vi "nanocal -- generate 3D curvature ellipsoid --  V5.vi"(0 "parameter keys IN":T2[](array[typedef])=[enum."ζ", enum."τ1", enum."τS", enum."τN", enum."τC", enum."κ0"], 5 "parameter tensor order IN":map{i32, T2}(c390), 7 "parameters IN":map{T2, dbl}(c390), 9 "data IN":T3={"dz/dω  (sec/rad)"=[], "z "=[1.7183506006211996e-05-0.0001154032788780638i, 1.7124360968751133e-05-0.0001154114779288915i, 1.7049104347380084e-05-0.00011541542942613611i, 1.700437896335042e-05-0.00011541749156201827i, 1.6984579723285106e-05-0.00011542204741013496i, 1.702277369054923e-05-0.00011543195548892015i, 1.713094025845651e-05-0.00011543928112855599i, 1.734249707866828e-05-0.00011543960094139092i, 1.768320429215342e-05-0.0001154245402225022i, 1.8195281152538477e-05-0.00011538335923575508i, 1.8917228661806973e-05-0.00011530288392402138i, 1.9897834564883332e-05-0.00011516640933089982i, 2.154104046962704e-05-0.0001148906117047364i, 2.3247799321765792e-05-0.00011455940834964969i, 2.5364678450551808e-05-0.00011410149936074356i, 2.8645788781885885e-05-0.00011331572480450341i, 3.204749554800641e-05-0.00011242961468546203i, 3.783559691555022e-05-0.00011080033368711338i, 4.245015867332296e-05-0.00010941815048749576i, 4.909131821431355e-05-0.0001073312840925185i, 5.511821898441184e-05-0.00010535829212367013i, 6.178843506022867e-05-0.00010310289174359778i, 7.1079604965352e-05-9.985157907779013e-05i, 7.922304381453334e-05-9.690255343156676e-05i, 8.814778883893872e-05-9.35627973091444e-05i, 9.806709148886077e-05-8.971246458508318e-05i, 0.00011119043245647465-8.437841897470898e-05i, 0.00012253184919712196-7.953180105990741e-05i, 0.00013777724317049346-7.26422052575784e-05i, 0.0001508081004573332-6.638511645494567e-05i, 0.00016547294918783876-5.890291826790314e-05i, 0.00018003847596605868-5.097295421607585e-05i, 0.00019518361086534857-4.2160672625888326e-05i, 0.00021134179818259658-3.207632261667366e-05i, 0.0002372041782935464-1.434566976209705e-05i, 0.00025518143132024254-7.65423157605567e-07i, 0.0002835129702467886+2.297908707067173e-05i, 0.0003060118087631287+4.414715126576145e-05i, 0.00032860772064336976+6.780161699354136e-05i, 0.0003492674091322389+9.188627597766353e-05i, 0.00037498324855458583+0.0001258445655672888i, 0.00040021078021115026+0.00016463936720210011i, 0.00041969942568205823+0.0001996255883353531i, 0.00044367338947118773+0.00025154867300893595i, 0.0004634793607238068+0.0003068834938295352i, 0.00047921028781215815+0.00036805191402776324i, 0.0004880906353641744+0.00042166295770603194i, 0.0004932212623741357+0.0004947057496862386i, 0.000491476456593048+0.0005562791342814882i, 0.000480893803992059+0.0006363872629062725i, 0.0004535995818650303+0.0007373086546111893i, 0.000417087772881063+0.0008226852134031236i, 0.0003564148692854789+0.0009214817173403453i, 0.0003049201646356487+0.0009841224100520793i, 0.00021260191240459413+0.0010684135492785532i, 0.00011714858948470126+0.001130293664798013i, 1.675457544365132e-05+0.0011752384955043165i, -6.8674075405897e-05+0.0012001399159748158i, -0.000156473047607305+0.0012143601357779102i, -0.00026709373934749337+0.0012167952520739987i, -0.0003544271565676041+0.001206585218500233i, -0.00047937600197311275+0.0011721904461218277i, -0.0006086290582260493+0.0011080263068835828i, -0.0007031877411848573+0.0010369948237613604i, -0.0007564526901441745+0.0009845652865779295i, -0.000802489180995596+0.0009292050493656664i, -0.0008414596018105983+0.0008721985101652608i, -0.0008809346482248761+0.0008000538120167723i, -0.0009073902840241921+0.0007382113118499092i, -0.0009264953054508651+0.000680980624166274i, -0.0009405659412141811+0.0006247883223244968i, -0.000951649722530156+0.0005564170049287236i, -0.0009557485581057351+0.0005027508202624884i, -0.0009558464741053665+0.0004515634249715623i, -0.0009509110176922098+0.0003899637122391104i, -0.0009411315169847015+0.00033238768338539245i, -0.0009303400913929496+0.0002890952314710416i, -0.0009171113529290538+0.00024772942260094455i, -0.0009022111527275027+0.00020961974320628598i, -0.0008813746494947608+0.00016554205395646727i, -0.0008581837971946129+0.00012481593212717478i, -0.0008372063466683705+9.328565348151487e-05i, -0.0008165626610594428+6.595676342721183e-05i, -0.0007901155435838691+3.51376371228606e-05i, -0.0007682834352800848+1.2585785624721776e-05i, -0.000746231015527196-7.956667433689733e-06i, -0.0007238798463130141-2.6771164006128246e-05i, -0.0007015567569177018-4.3779400880525094e-05i, -0.000679301954671598-5.9154880569231366e-05i, -0.0006572001413831251-7.301304884663801e-05i, -0.000629855254567978-8.838260380910578e-05i, -0.0006083942229188815-9.917719243438264e-05i, -0.0005768631156754208-0.00011317657292622015i, -0.0005562177438951648-0.00012121832857134644i, -0.0005359092039599222-0.00012831021292074535i, -0.0005145186443378148-0.00013494179211461784i, -0.0004951602053444319-0.00014023403510992087i, -0.00047624970229075174-0.00014478034103386663i, -0.0004577401041527736-0.00014865456703421655i, -0.00043519037796120065-0.00015262867452433312i], "ω (rad/sec)"=[32012.991918577427, 32390.261658505893, 32466.39798177853, 32499.14340521798, 32517.39286113775, 32529.046092051318, 32537.14525712326, 32543.111142615544, 32547.696343954158, 32551.33675949651, 32554.302325209504, 32556.769142360055, 32558.856995237307, 32560.650202739795, 32562.209843476354, 32563.58125099723, 32564.7987833122, 32565.88895894197, 32566.872575330308, 32567.766175404246, 32568.583086316496, 32569.334166794306, 32570.02835688638, 32570.673085530187, 32571.274580490695, 32571.838104118455, 32572.36813539066, 32572.868514009202, 32573.342552524307, 32573.793126289274, 32574.222746575288, 32574.633618125405, 32575.027687968828, 32575.40668442971, 32575.772149741057, 32576.12546690325, 32576.467883345118, 32576.800529469096, 32577.124435064776, 32577.440543590797, 32577.749724325146, 32578.052781957467, 32578.35046682089, 32578.643482565894, 32578.932492128843, 32579.218126471686, 32579.500987779396, 32579.781656707495, 32580.06069600583, 32580.338656060805, 32580.616078519142, 32580.89350097748, 32581.171461032456, 32581.45050033079, 32581.73116925889, 32582.0140305666, 32582.29966469628, 32582.58867447239, 32582.88169000423, 32583.179375080817, 32583.48243271314, 32583.791613234323, 32584.10772197351, 32584.43162756919, 32584.764273480003, 32585.106690135035, 32585.460007297228, 32585.825472395412, 32586.204468856296, 32586.59853891288, 32587.009410462997, 32587.439030535847, 32587.889604513977, 32588.363642815923, 32588.86402143446, 32589.39405291983, 32589.957576334426, 32590.559071508098, 32591.203800151903, 32591.897990030815, 32592.64907072179, 32593.46598163404, 32594.359581707977, 32595.343197883154, 32596.433373726086, 32597.650906041054, 32599.022313348767, 32600.58195429849, 32602.375161800977, 32604.46301467823, 32606.929831615616, 32609.895397541775, 32613.535812870963, 32618.12101442274, 32624.086899701866, 32632.186064986967, 32643.839295900536, 32662.088751820305, 32694.834175046595, 32770.97049853239]}, 11 "errors IN":T1={"one"=enum."τ1", "two"=enum."τS", "sigmaone"=enum."στ1", "sigmatwo"=enum."στS", "three"=enum."τN", "sigmathree"=enum."στN", "pars & errors"={}, "T22 factor"=5.0, "CN2 factor"=0.1, "δG/G"=0.5535743588970453, "noise T"=0.1, "Δlogs"=[3.0, 1.0], "Δlog ηs"=[4.618033988749895, 2.381966011250105]} {"Δlog ηs" format="%#_2f"; "Δlogs" format="%#_2f"; "noise T" format="%#_3f"; "δG/G" format="%#_3f"; "CN2 factor" min=0.0 max=0.3 step=1e-06 scale=0.01..1.0 scale format="%#_2f"; "T22 factor" min=0.0 max=0.3 step=1e-06 scale=0.1..20.0 scale format="%#_2f"}, 12 "newton parameters":T4={"method"=enum."ignore", "weighting"=enum."dω √(|dz/dω|)", "PID-P"=0.009761510697263134, "PID-I"=5} {"PID-P" scale=1e-09..10.0 scale format="%#_3p"}) -> (15 "errors pair OUT":T1={"one"=enum."τ1", "two"=enum."τS", "sigmaone"=enum."στ1", "sigmatwo"=enum."στS", "three"=enum."τN", "sigmathree"=enum."στN", "pars & errors"={}, "T22 factor"=5.0, "CN2 factor"=0.1, "δG/G"=0.5535743588970453, "noise T"=0.1, "Δlogs"=[3.0, 1.0], "Δlog ηs"=[4.618033988749895, 2.381966011250105]} {"Δlog ηs" format="%#_2f"; "Δlogs" format="%#_2f"; "noise T" format="%#_3f"; "δG/G" format="%#_3f"; "CN2 factor" min=0.0 max=0.3 step=1e-06 scale=0.01..1.0 scale format="%#_2f"; "T22 factor" min=0.0 max=0.3 step=1e-06 scale=0.1..20.0 scale format="%#_2f"})   [LabVIEW 2021]
uses:
  3-lorentzian-parameters.ctl
  nanocal -- gradient descent -- parameters.ctl
  linear regression type.ctl
  nanocal-goodness-weighting-strategy.ctl
  nanocal -- gradient descent-- data.ctl
  3D curvature triplet control -- V2.ctl
  nanocal generate curvature ellipse -- action.ctl
  3-lorentzian-heat-response action.ctl
  array -- 3-finitediff.vi
  5-lorentzian-heat-response -- analytic derivatives -- grad and curvature -- V6.vi
  <vilib>/Analysis/Matrix/Numeric/Conversions/Array To Matrix.vi
  <vilib>/Analysis/Matrix/Numeric/Conversions/Array To Matrix - RA2.vi
  <vilib>/Analysis/baseanly.llb/Inverse Matrix.vi
  <vilib>/Analysis/baseanly.llb/Real Inverse Matrix.vi
  <vilib>/Analysis/Matrix/Numeric/Conversions/Matrix To Array.vi
  <vilib>/Analysis/Matrix/Numeric/Conversions/Matrix To Array - RM.vi
  <vilib>/Analysis/Matrix/Numeric/Conversions/Array To Matrix - RA.vi
  <vilib>/Analysis/7linalg.llb/Solve Linear Equations.vi
  <vilib>/Analysis/7linalg.llb/Solve Linear Equations (multiple right hand).vi
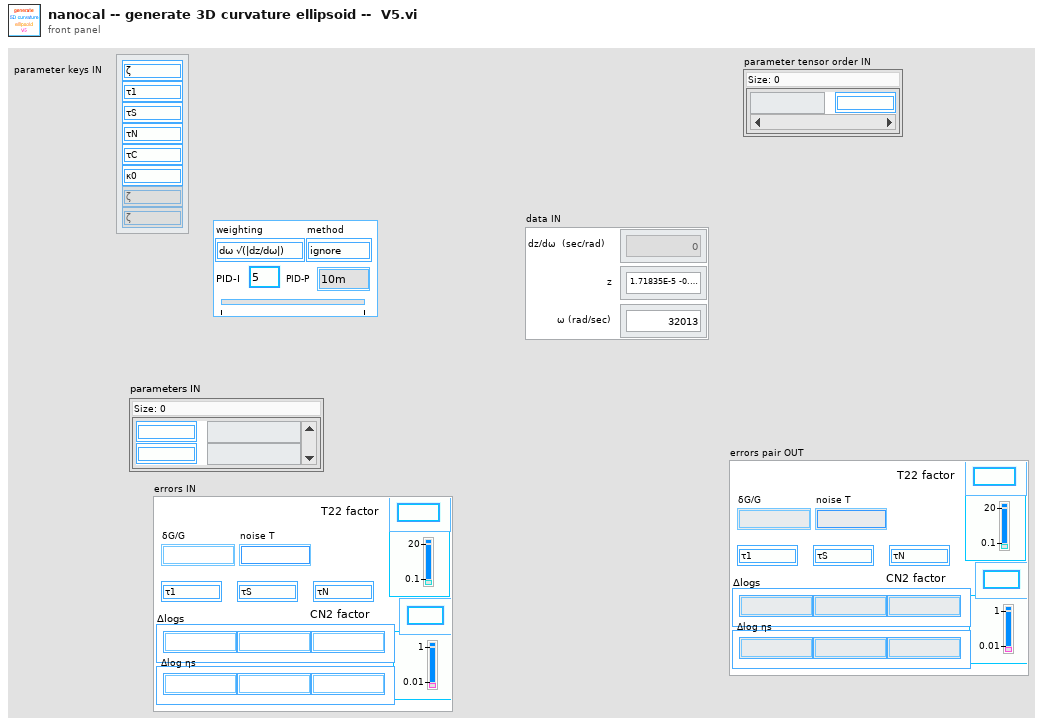
[diagram p1: front panel]
types:
  T1 = typedef "3D curvature triplet control -- V2.ctl" = cluster{"one":T2, "two":T2, "sigmaone":T2, "sigmatwo":T2, "three":T2, "sigmathree":T2, "pars & errors":map{T2, dbl}, "T22 factor":dbl, "CN2 factor":dbl, "δG/G":dbl, "noise T":dbl, "Δlogs":dbl[], "Δlog ηs":dbl[]}
  T2 = typedef "3-lorentzian-parameters.ctl" = enum16{"ζ", "τ1", "τS", "τN", "τC", "κ0", "m1", "m2", "m3", "T (K)", "B (T)", "θ (deg)", "side (S|R)", "set of (B|T)", "Re(offset)", "Im(offset)", "στ1", "στ1-", "στ1+", "στS", "στS-", "στS+", "στN", "στN-", "στN+", "τ11", "τ12", "τ21", "τ22", "τN1", "τN2", "σηlogτ1", "σηlogτS", "σηlogτN", "σlogτ1", "σlogτS", "σlogτN", "σητ1", "σητS", "σητN", "noiseT"}
  T3 = typedef "nanocal -- gradient descent-- data.ctl" = cluster{"dz/dω  (sec/rad)":cdb[], "z ":cdb[], "ω (rad/sec)":dbl[]}
  T4 = typedef "nanocal -- gradient descent -- parameters.ctl" = cluster{"method":T5, "weighting":T6, "PID-P":dbl, "PID-I":i32}
  T5 = typedef "linear regression type.ctl" = enum16{"ignore", "gradient", "newton"}
  T6 = typedef "nanocal-goodness-weighting-strategy.ctl" = enum16{"dω", "dω √(|dz/dω|)", "dω |dz/dω|", "phase", "andreas", "sum", "anti-andr", "ark"}
  T7 = typedef "nanocal generate curvature ellipse -- action.ctl" = enum16{"errors-log", "errors-linear"}
  T8 = typedef "3-lorentzian-heat-response action.ctl" = enum16{"calc R", "create string", "calc m1m2m3", "dζ", "dT1", "dτS", "dτN", "dτC", "d-all", "dκ0", "T(K)", "m1", "m2", "m3", "parse string", "θ (deg)", "B (T)", "onlygrads", "newton", "create emty string", "simple2nd", "calc R2", "ScalarProd", "ScalarProd-diff", "nothing", "ScalarProd-eta", "tolog", "ignore", "three2nd", "eta-errors"}
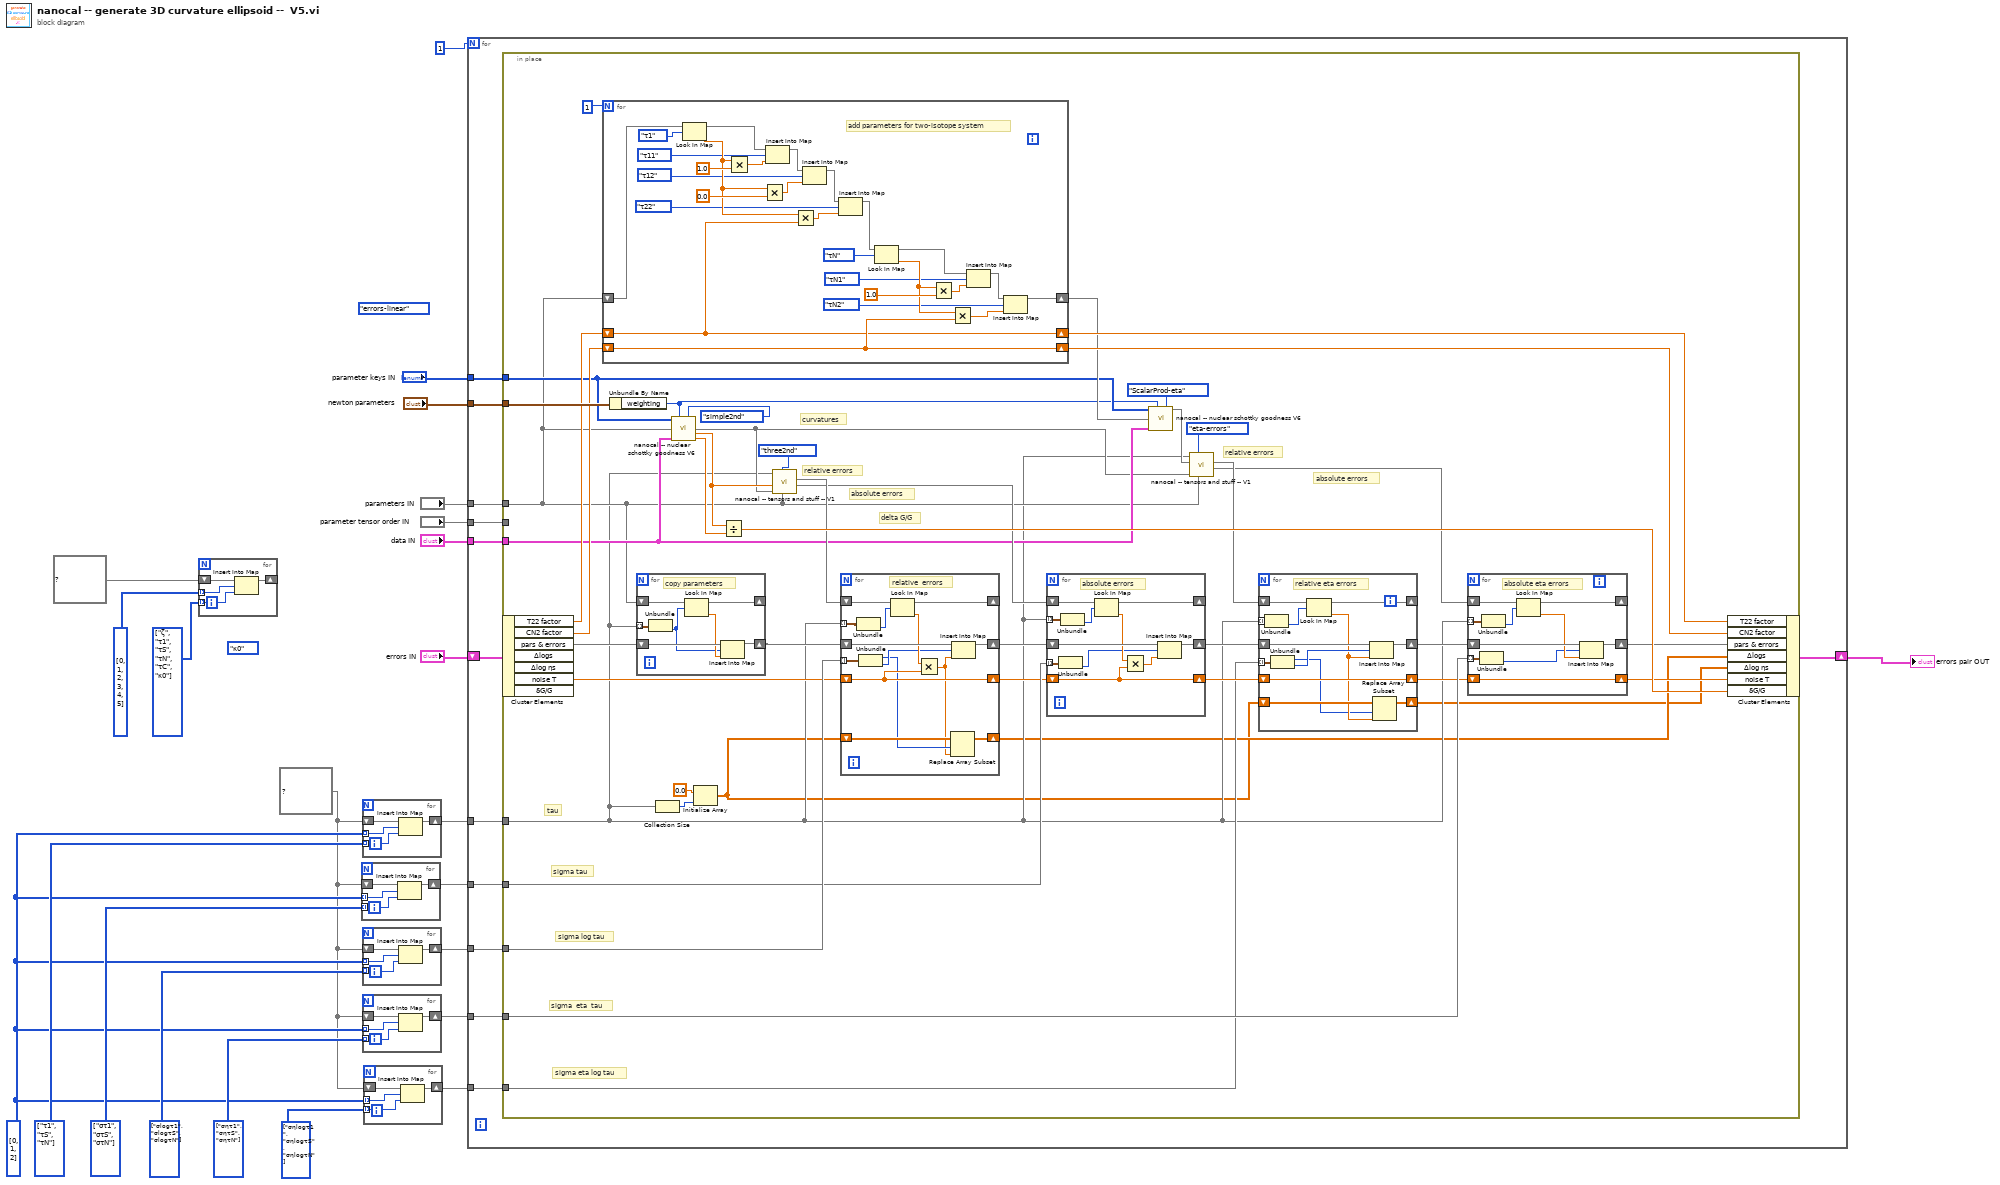
[diagram p0: block diagram]
diagram:
  w4 = T2[] [enum."σηlogτ1", enum."σηlogτS", enum."σηlogτN"] items=["ζ", "τ1", "τS", "τN", "τC", "κ0", "m1", "m2", "m3", "T (K)", "B (T)", "θ (deg)", "side (S|R)", "set of (B|T)", "Re(offset)", "Im(offset)", "στ1", "στ1-", "στ1+", "στS", "στS-", "στS+", "στN", "στN-", "στN+", "τ11", "τ12", "τ21", "τ22", "τN1", "τN2", "σηlogτ1", "σηlogτS", "σηlogτN", "σlogτ1", "σlogτS", "σlogτN", "σητ1", "σητS", "σητN", "noiseT"]
  w9 = T2[] [enum."σlogτ1", enum."σlogτS", enum."σlogτN"] items=["ζ", "τ1", "τS", "τN", "τC", "κ0", "m1", "m2", "m3", "T (K)", "B (T)", "θ (deg)", "side (S|R)", "set of (B|T)", "Re(offset)", "Im(offset)", "στ1", "στ1-", "στ1+", "στS", "στS-", "στS+", "στN", "στN-", "στN+", "τ11", "τ12", "τ21", "τ22", "τN1", "τN2", "σηlogτ1", "σηlogτS", "σηlogτN", "σlogτ1", "σlogτS", "σlogτN", "σητ1", "σητS", "σητN", "noiseT"]
  w10 = T2[] [enum."σητ1", enum."σητS", enum."σητN"] items=["ζ", "τ1", "τS", "τN", "τC", "κ0", "m1", "m2", "m3", "T (K)", "B (T)", "θ (deg)", "side (S|R)", "set of (B|T)", "Re(offset)", "Im(offset)", "στ1", "στ1-", "στ1+", "στS", "στS-", "στS+", "στN", "στN-", "στN+", "τ11", "τ12", "τ21", "τ22", "τN1", "τN2", "σηlogτ1", "σηlogτS", "σηlogτN", "σlogτ1", "σlogτS", "σlogτN", "σητ1", "σητS", "σητN", "noiseT"]
  w11 = T2[] [enum."στ1", enum."στS", enum."στN"] items=["ζ", "τ1", "τS", "τN", "τC", "κ0", "m1", "m2", "m3", "T (K)", "B (T)", "θ (deg)", "side (S|R)", "set of (B|T)", "Re(offset)", "Im(offset)", "στ1", "στ1-", "στ1+", "στS", "στS-", "στS+", "στN", "στN-", "στN+", "τ11", "τ12", "τ21", "τ22", "τN1", "τN2", "σηlogτ1", "σηlogτS", "σηlogτN", "σlogτ1", "σlogτS", "σlogτN", "σητ1", "σητS", "σητN", "noiseT"]
  (unwired) 3-lorentzian-parameters."κ0" ("X selector")
  w3 = i32[] [0, 1, 2]
  w2 = map{i32, T2} {} ("parameters IN")
  w13 = T2[] [enum."τ1", enum."τS", enum."τN"] items=["ζ", "τ1", "τS", "τN", "τC", "κ0", "m1", "m2", "m3", "T (K)", "B (T)", "θ (deg)", "side (S|R)", "set of (B|T)", "Re(offset)", "Im(offset)", "στ1", "στ1-", "στ1+", "στS", "στS-", "στS+", "στN", "στN-", "στN+", "τ11", "τ12", "τ21", "τ22", "τN1", "τN2", "σηlogτ1", "σηlogτS", "σηlogτN", "σlogτ1", "σlogτS", "σlogτN", "σητ1", "σητS", "σητN", "noiseT"]
  w16 = T2[] [enum."ζ", enum."τ1", enum."τS", enum."τN", enum."τC", enum."κ0"] items=["ζ", "τ1", "τS", "τN", "τC", "κ0", "m1", "m2", "m3", "T (K)", "B (T)", "θ (deg)", "side (S|R)", "set of (B|T)", "Re(offset)", "Im(offset)", "στ1", "στ1-", "στ1+", "στS", "στS-", "στS+", "στN", "στN-", "στN+", "τ11", "τ12", "τ21", "τ22", "τN1", "τN2", "σηlogτ1", "σηlogτS", "σηlogτN", "σlogτ1", "σlogτS", "σlogτN", "σητ1", "σητS", "σητN", "noiseT"]
  (unwired) nanocal_generate_curvature_ellipse_--_action."errors-linear" ("Enum")
  n1 = for {
    tunnel: w16 -> [w24] mode=indexing
    shift-right: [w26] -> _
    shift-left: map{i32, T2} {} ("parameters IN") -> [w27]
    tunnel: i32[] [0, 1, 2, 3, 4, 5] -> [w25] mode=indexing
    n2 = Insert Into Map(map in=w27, key=w25, value=w24) -> (map out=w26:map{i32, T2})  [unwired: 2 out]
  }
  n3 = for {
    tunnel: w11 -> [w28] mode=indexing
    shift-right: [w30] -> w7
    shift-left: w2 -> [w31]
    tunnel: w3 -> [w29] mode=indexing
    n4 = Insert Into Map(map in=w31, key=w29, value=w28) -> (map out=w30:map{i32, T2})  [unwired: 2 out]
  }
  n5 = for {
    tunnel: w13 -> [w32] mode=indexing
    shift-right: [w34] -> w12
    shift-left: w2 -> [w35]
    tunnel: w3 -> [w33] mode=indexing
    n6 = Insert Into Map(map in=w35, key=w33, value=w32) -> (map out=w34:map{i32, T2})  [unwired: 2 out]
  }
  n7 = for {
    tunnel: w9 -> [w36] mode=indexing
    shift-right: [w38] -> w8
    shift-left: w2 -> [w39]
    tunnel: w3 -> [w37] mode=indexing
    n8 = Insert Into Map(map in=w39, key=w37, value=w36) -> (map out=w38:map{i32, T2})  [unwired: 2 out]
  }
  n9 = for {
    tunnel: w10 -> [w40] mode=indexing
    shift-right: [w42] -> w6
    shift-left: w2 -> [w43]
    tunnel: w3 -> [w41] mode=indexing
    n10 = Insert Into Map(map in=w43, key=w41, value=w40) -> (map out=w42:map{i32, T2})  [unwired: 2 out]
  }
  n11 = for {
    tunnel: w4 -> [w44] mode=indexing
    shift-right: [w46] -> w1
    shift-left: w2 -> [w47]
    tunnel: w3 -> [w45] mode=indexing
    n12 = Insert Into Map(map in=w47, key=w45, value=w44) -> (map out=w46:map{i32, T2})  [unwired: 2 out]
  }
  n13 = for {
    N: 1 -> [_]
    tunnel: "newton parameters" -> [w59]
    tunnel: "data IN" -> [w58]
    tunnel: "parameters IN" -> [w57]
    tunnel: "parameter keys IN" -> [w56]
    tunnel: "parameter tensor order IN" -> [w55]
    shift-right: [w49] -> w5
    shift-left: "errors IN" -> [w54]
    tunnel: w12 -> [w53]
    tunnel: w8 -> [w52]
    tunnel: w7 -> [w51]
    tunnel: w6 -> [w50]
    tunnel: w1 -> [w48]
    n14 = in-place {
      in-place-border: w59 -> [w104]
      in-place-border: w58 -> [w75]
      in-place-border: w57 -> [w73]
      in-place-border: w56 -> [w92]
      in-place-border: w55 -> [_]
      in-place-border: w53 -> [w63]
      in-place-border: w52 -> [w85]
      in-place-border: w51 -> [w81]
      in-place-border: w50 -> [w69]
      in-place-border: w48 -> [w68]
      # "sigma eta log tau"
      # "curvatures"
      # "sigma log tau"
      # "sigma  eta  tau"
      # "sigma tau"
      # "tau"
      # "relative errors"
      # "absolute errors"
      # "delta G/G"
      # "relative errors"
      # "absolute errors"
      n15 = in-place-cluster #1(w54) -> ("T22 factor"=w101:dbl, "CN2 factor"=w99:dbl, "pars & errors"=w87:map{T2, dbl}, "noise T"=w80:dbl)  [unwired: 3 out]
      n16 = for {
        N: 1 -> [_]
        shift-right: [w157] -> w93
        shift-left: w73 -> [w174]
        shift-right: [w155] -> w98
        shift-left: w101 -> [w155]
        shift-right: [w156] -> w97
        shift-left: w99 -> [w156]
        # "add parameters for two-isotope system"
        n17 = Look In Map(map=w174, key=3-lorentzian-parameters."τ1" ("X selector")) -> (value=w175:dbl)  [unwired: 1 in, 1 out]
        n18 = Multiply(x=w175, y=1.0) -> (x*y=w172:dbl)
        n19 = Multiply(x=w175, y=0.0 ("value")) -> (x*y=w169:dbl)
        n20 = Insert Into Map(map in=w174, key=3-lorentzian-parameters."τ11" ("X selector"), value=w172) -> (map out=w171:map{T2, dbl})  [unwired: 2 out]
        n21 = Multiply(x=w175, y=w155) -> (x*y=w166:dbl)
        n22 = Insert Into Map(map in=w171, key=3-lorentzian-parameters."τ12" ("X selector"), value=w169) -> (map out=w168:map{T2, dbl})  [unwired: 2 out]
        n23 = Insert Into Map(map in=w168, key=3-lorentzian-parameters."τ22" ("X selector"), value=w166) -> (map out=w163:map{T2, dbl})  [unwired: 2 out]
        n24 = Look In Map(map=w163, key=3-lorentzian-parameters."τN" ("X selector")) -> (value=w164:dbl)  [unwired: 1 in, 1 out]
        n25 = Multiply(x=w164, y=1.0) -> (x*y=w162:dbl)
        n26 = Multiply(x=w164, y=w156) -> (x*y=w158:dbl)
        n27 = Insert Into Map(map in=w163, key=3-lorentzian-parameters."τN1" ("X selector"), value=w162) -> (map out=w160:map{T2, dbl})  [unwired: 2 out]
        n28 = Insert Into Map(map in=w160, key=3-lorentzian-parameters."τN2" ("X selector"), value=w158) -> (map out=w157:map{T2, dbl})  [unwired: 2 out]
      }
      n29 = Unbundle By Name(w104) -> ("weighting"=w91:T6)
      n30 = for {
        shift-right: [w151] -> _
        shift-left: w73 -> [w151]
        tunnel: w63 -> [w154] mode=indexing
        shift-right: [w152] -> w84
        shift-left: w87 -> [w153]
        # "copy parameters"
        n31 = Unbundle(w154) -> ("X selector"=w149:T2)  [unwired: 1 out]
        n32 = Look In Map(map=w151, key=w149) -> (value=w150:dbl)  [unwired: 1 in, 1 out]
        n33 = Insert Into Map(map in=w153, key=w149, value=w150) -> (map out=w152:map{T2, dbl})  [unwired: 2 out]
      }
      n34 = Collection Size(1:w63) -> (0:w64:i32)
      n35 = call "nanocal -- nuclear schottky goodness V6.vi"("parameter keys  IN"=w92, "weighting strategy"=w91, "action"=3-lorentzian-heat-response_action."simple2nd", "parameters IN"=w73, "data"=w75) -> ("⟨ λ1 dξ(ω)/dλ1 | λ2 dξ(ω)/dλ2 ⟩"=w74:map{T2[], dbl}, "G = ⟨ξ(ω)|ξ(ω)⟩"=w90:dbl, "⟨ζ(ω)|ζ(ω)⟩"=w89:dbl)  [unwired: 6 in, 2 out]
      n36 = Initialize Array(0.0 ("element"), w64) -> (w61:dbl[])
      n37 = Divide(x=w90, y=w89) -> (x/y=w88:dbl)
      n38 = call "nanocal -- tensors and stuff -- V1.vi"("parameters IN"=w73, "action"=3-lorentzian-heat-response_action."three2nd", "d2G / d log λ1 d log λ2  = ⟨ λ1 dζ(ω)/dλ1 | λ2 dζ(ω)/dλ2 ⟩"=w74, "G"=w90, "parameter tensor order IN"=w63) -> ("map absolute out"=w82:map{T2, dbl}, "map relative out"=w86:map{T2, dbl})  [unwired: 4 in, 1 out]
      n39 = for {
        shift-right: [w145] -> _
        shift-left: w86 -> [w145]
        tunnel: w85 -> [w148] mode=indexing
        shift-right: [w146] -> w83
        shift-left: w84 -> [w147]
        shift-right: [w143] -> w79
        shift-left: w80 -> [w143]
        tunnel: w63 -> [w142] mode=indexing
        shift-right: [w138] -> w62
        shift-left: w61 -> [w139]
        # "relative  errors"
        n40 = Unbundle(w142) -> ("X selector"=w141:T2)  [unwired: 1 out]
        n41 = Unbundle(w148) -> ("index"=w137:i32, "X selector"=w140:T2)
        n42 = Look In Map(map=w145, key=w141) -> (value=w144:dbl)  [unwired: 1 in, 1 out]
        n43 = Multiply(x=w144, y=w143) -> (x*y=w136:dbl)
        n44 = Replace Array Subset(array=w139, new element=w136, index=w137) -> (w138:dbl[])
        n45 = Insert Into Map(map in=w147, key=w140, value=w136) -> (map out=w146:map{T2, dbl})  [unwired: 2 out]
      }
      n46 = for {
        shift-right: [w132] -> _
        shift-left: w82 -> [w132]
        tunnel: w81 -> [w135] mode=indexing
        shift-right: [w133] -> w78
        shift-left: w83 -> [w134]
        shift-right: [w129] -> w76
        shift-left: w79 -> [w129]
        tunnel: w63 -> [w127] mode=indexing
        # "absolute errors"
        n47 = Unbundle(w135) -> ("X selector"=w128:T2)  [unwired: 1 out]
        n48 = Unbundle(w127) -> ("X selector"=w126:T2)  [unwired: 1 out]
        n49 = Look In Map(map=w132, key=w126) -> (value=w131:dbl)  [unwired: 1 in, 1 out]
        n50 = Multiply(x=w131, y=w129) -> (x*y=w130:dbl)
        n51 = Insert Into Map(map in=w134, key=w128, value=w130) -> (map out=w133:map{T2, dbl})  [unwired: 2 out]
      }
      n52 = call "nanocal -- nuclear schottky goodness V6.vi"("parameter keys  IN"=w92, "weighting strategy"=w91, "action"=3-lorentzian-heat-response_action."ScalarProd-eta", "parameters IN"=w93, "data"=w75) -> ("dG / dlog λ  =  ⟨ξ(ω) | λdζ(ω)/dλ ⟩"=w94:map{T2, dbl})  [unwired: 6 in, 4 out]
      n53 = call "nanocal -- tensors and stuff -- V1.vi"("parameters IN"=w73, "action"=3-lorentzian-heat-response_action."eta-errors", "d2G / d log λ1 d log λ2  = ⟨ λ1 dζ(ω)/dλ1 | λ2 dζ(ω)/dλ2 ⟩"=w74, "dG / dlog λ  =  ⟨ (ξ(ω)-ζ(ω)) | λdζ(ω)/dλ ⟩"=w94, "parameter tensor order IN"=w63) -> ("map absolute out"=w70:map{T2, dbl}, "map relative out"=w77:map{T2, dbl})  [unwired: 4 in, 1 out]
      n54 = for {
        shift-right: [w122] -> _
        shift-left: w77 -> [w122]
        tunnel: w68 -> [w125] mode=indexing
        shift-right: [w123] -> w72
        shift-left: w78 -> [w124]
        shift-right: [w121] -> w67
        shift-left: w76 -> [w121]
        tunnel: w63 -> [w119] mode=indexing
        shift-right: [w116] -> w60
        shift-left: w61 -> [w117]
        # "relative eta errors"
        n55 = Unbundle(w119) -> ("X selector"=w118:T2)  [unwired: 1 out]
        n56 = Unbundle(w125) -> ("index"=w114:i32, "X selector"=w120:T2)
        n57 = Look In Map(map=w122, key=w118) -> (value=w115:dbl)  [unwired: 1 in, 1 out]
        n58 = Insert Into Map(map in=w124, key=w120, value=w115) -> (map out=w123:map{T2, dbl})  [unwired: 2 out]
        n59 = Replace Array Subset(array=w117, new element=w115, index=w114) -> (w116:dbl[])
      }
      n60 = for {
        shift-right: [w111] -> _
        shift-left: w70 -> [w111]
        shift-right: [w112] -> w71
        shift-left: w72 -> [w113]
        shift-right: [w110] -> w66
        shift-left: w67 -> [w110]
        tunnel: w63 -> [w108] mode=indexing
        tunnel: w69 -> [w106] mode=indexing
        # "absolute eta errors"
        n61 = Unbundle(w106) -> ("X selector"=w105:T2)  [unwired: 1 out]
        n62 = Unbundle(w108) -> ("X selector"=w107:T2)  [unwired: 1 out]
        n63 = Look In Map(map=w111, key=w107) -> (value=w109:dbl)  [unwired: 1 in, 1 out]
        n64 = Insert Into Map(map in=w113, key=w105, value=w109) -> (map out=w112:map{T2, dbl})  [unwired: 2 out]
      }
      n65 = in-place-cluster #1("T22 factor"=w98, "CN2 factor"=w97, "pars & errors"=w71, "Δlogs"=w62, "Δlog ηs"=w60, "noise T"=w66, "δG/G"=w88) -> (w49:T1)
    }
  }
  "errors pair OUT" <- w5
